vi "Check Status.vi"(8 "error in (no error)":errorcluster, 11 "Spectrometer iHR320 in":refnum<class "Spectrometer iHR320.lvclass">) -> (0 "error out":errorcluster, 1 "Status":string, 2 "Ready?":bool, 3 "Spectrometer iHR320 out":refnum<class "Spectrometer iHR320.lvclass">)   [LabVIEW 2009, in "Spectrometer iHR320.lvclass"]
doc: "(Dynamic) Check if the instrument is powered on and update its member fields with the instrument's current status. Optionally return a text status message."
uses:
  Spectrometer iHR320.lvclass
  Utility Classes/Scannable/Scannable.lvclass
  Spectrometer iHR320.lvclass/Spectrometer iHR320.ctl
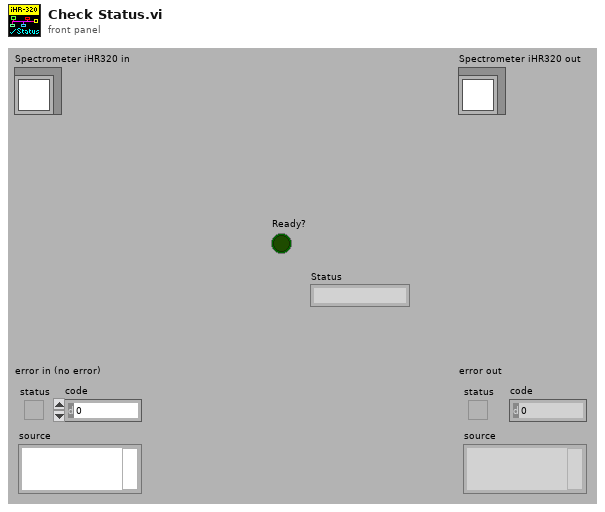
[diagram p1: front panel]
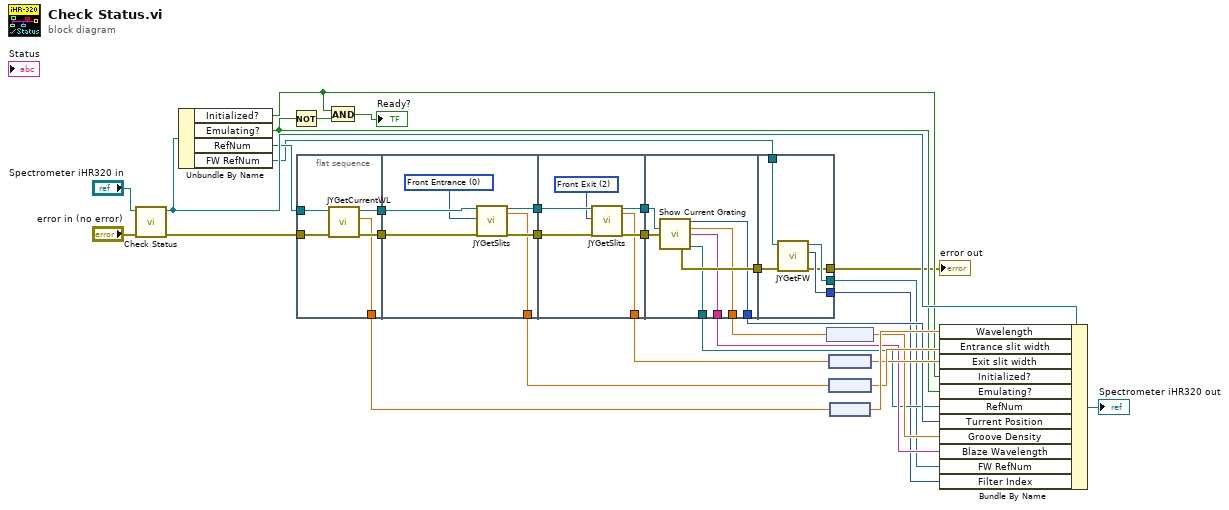
[diagram p0: block diagram]
diagram:
  n1 = call-parent "Check Status.vi"("error in (no error)"="error in (no error)", "Instrument in"="Spectrometer iHR320 in") -> ("error out"=w19:errorcluster, "Instrument out"=w30:refnum<class "Spectrometer iHR320.lvclass">)  [unwired: 6 in, 2 out]
  n2 = Unbundle By Name(w30) -> ("Initialized?"=w21:bool, "Emulating?"=w22:bool, "RefNum"=w20:refnum<k7>, "FW RefNum"=w11:refnum<k7>)
  n3 = Not(x=w22) -> (.not. x?=w23:bool)
  n4 = flat-sequence {
    tunnel: w20 -> [w37]
    tunnel: w19 -> [w36]
    tunnel: [w35] -> w18
    tunnel: [w34] -> w15
    tunnel: [w33] -> w10
    tunnel: w18 -> [w43]
    tunnel: [w42] -> w17
    tunnel: w15 -> [w41]
    tunnel: [w40] -> w14
    tunnel: [w39] -> w9
    tunnel: w17 -> [w49]
    tunnel: [w48] -> w16
    tunnel: w14 -> [w47]
    tunnel: [w46] -> w13
    tunnel: [w45] -> w8
    tunnel: w16 -> [w56]
    tunnel: w13 -> [w55]
    tunnel: [w54] -> w12
    tunnel: [w53] -> w7
    tunnel: [w52] -> w6
    tunnel: [w51] -> w5
    tunnel: [w50] -> w4
    tunnel: w12 -> [w61]
    tunnel: w11 -> [w60]
    tunnel: [w59] -> w3
    tunnel: [w58] -> w2
    tunnel: [w57] -> w1
    frame #0 {
      n5 = call "JYGetCurrentWL.vi"("error in (no error)"=w36, "JYMONOLib.IJYMonoReqd In"=w37) -> ("error out"=w34:errorcluster, "Current WL"=w33:dbl, "JYMONOLib.IJYMonoReqd Out"=w35:refnum<k7>)  [unwired: 6 in, 1 out]
    }
    frame #1 {
      w38 = u16 0 items=["Front Entrance", "Side Entrance", "Front Exit", "Side Exit", "First Intermediate", "Second Intermediate"] ("Slit")
      n6 = call "JYGetSlits.vi"("MonoRefNum IN"=w43, "Slit"=w38, "error in (no error)"=w41) -> ("MonoRefNum Out"=w42:refnum<k7>, "Slit Width"=w39:dbl, "error out"=w40:errorcluster)  [unwired: 13 in, 1 out]
    }
    frame #2 {
      w44 = u16 2 items=["Front Entrance", "Side Entrance", "Front Exit", "Side Exit", "First Intermediate", "Second Intermediate"] ("Slit")
      n7 = call "JYGetSlits.vi"("MonoRefNum IN"=w49, "Slit"=w44, "error in (no error)"=w47) -> ("MonoRefNum Out"=w48:refnum<k7>, "Slit Width"=w45:dbl, "error out"=w46:errorcluster)  [unwired: 13 in, 1 out]
    }
    frame #3 {
      n8 = call "Show Current Grating.vi"("JYMONOLib.IJYMonoReqd  in"=w56, "error in (no error)"=w55) -> ("Grating Index"=w51:i32, "Current Grating"=w53:dbl, "Current Blaze"=w52:string, "error out"=w54:errorcluster, "JYMONOLib.IJYMonoReqd Out"=w50:refnum<k7>)  [unwired: 5 in, 4 out]
    }
    frame #4 {
      n9 = call "JYGetFW.vi"("error in (no error)"=w61, "FW RefNum In"=w60) -> ("error out"=w57:errorcluster, "Filter Index"=w58:i32, "FW RefNum Out"=w59:refnum<k7>)  [unwired: 7 in]
    }
  }
  n10 = And(x=w21, y=w23) -> (x .and. y?=→"Ready?":bool)
  n11 = node(w7) -> (w26:dbl[unit])
  n12 = node(w8) -> (w27:dbl[unit])
  n13 = node(w9) -> (w28:dbl[unit])
  n14 = node(w10) -> (w29:dbl[unit])
  n15 = Bundle By Name(cluster=w30, "Wavelength"=w29, "Entrance slit width"=w28, "Exit slit width"=w27, "Initialized?"=w21, "Emulating?"=w22, "RefNum"=w4, "Turrent Position"=w5, "Groove Density"=w26, "Blaze Wavelength"=w6, "FW RefNum"=w3, "Filter Index"=w2) -> (→"Spectrometer iHR320 out":refnum<class "Spectrometer iHR320.lvclass">)
  "error out" <- w1
